vi "testJob_Static_VI_Reference.vi"(10 "stdin":string) -> (2 "stdout":string)   [LabVIEW 2013, in "openCronJob.lvlib" / "Job.StaticVIRef.lvclass"]
uses:
  Job.StaticVIRef.lvclass
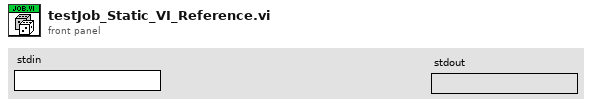
[diagram p1: front panel]
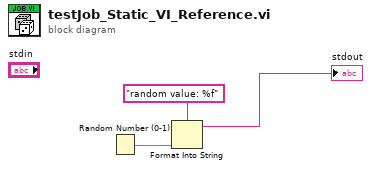
[diagram p0: block diagram]
diagram:
  n1 = Random Number (0-1)() -> (number: 0 to 1=w1:dbl)
  n2 = Format Into String(format string="random value: %f", w1) -> (resulting string=→"stdout":string)  [unwired: 2 in, 1 out]
